vi "Add Leaves.vi"(0 "TreeControl in":refnum<vi>, 1 "Relative File Path":string, 3 "FileName In Hierarchy?":bool, 5 "Tree Parent Tags":string[](array[string]), 7 "Tree Items Created In":variant, 9 "Group/Channel Names":string[](array[string]), 11 "error in (no error)":errorcluster) -> (8 "Tree Items Created Out":variant, 15 "error out":errorcluster)   [LabVIEW 2017, in "XTree.xctl"]
doc: "Adds channels to the tree at the last hierarchical level, if they don't already exist in the Tree Items Created variant."
uses:
  <vilib>/addons/_NIFileIO/XTree/XTree.xctl
panel:
  # "The Tree Parent Tags parameter's dimensions\ncorrespond to Group and Channel."
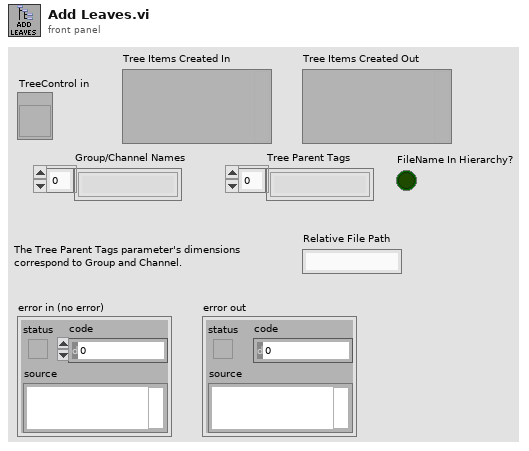
[diagram p1: front panel]
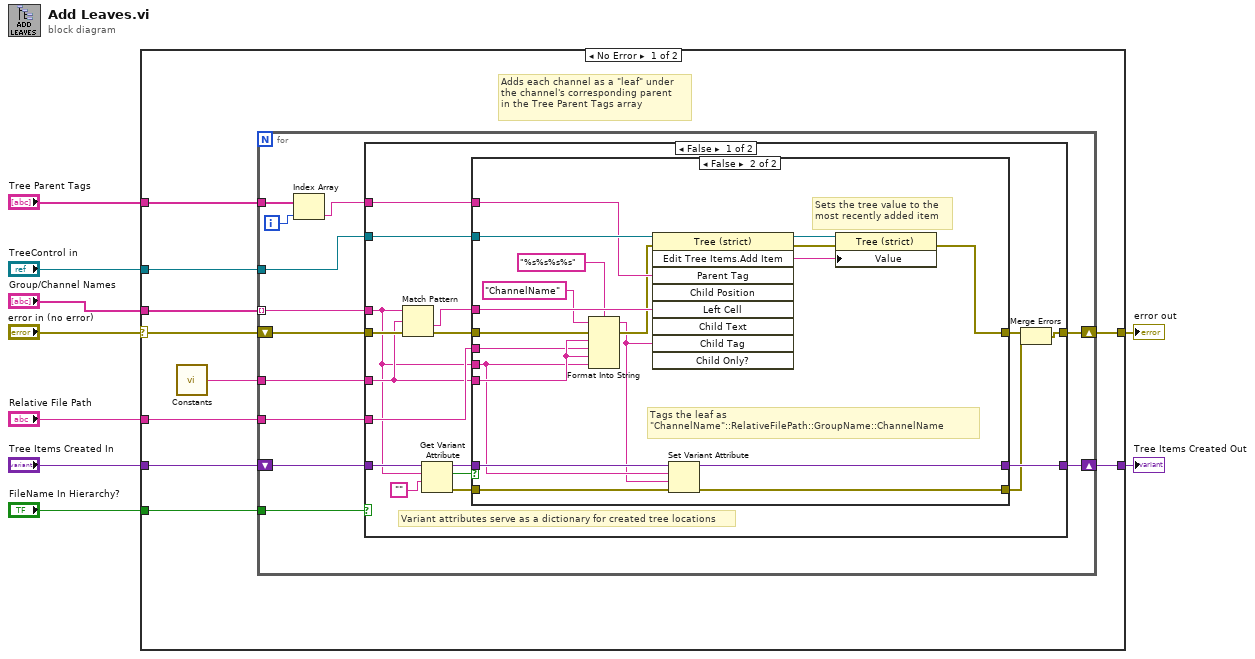
[diagram p0: block diagram]
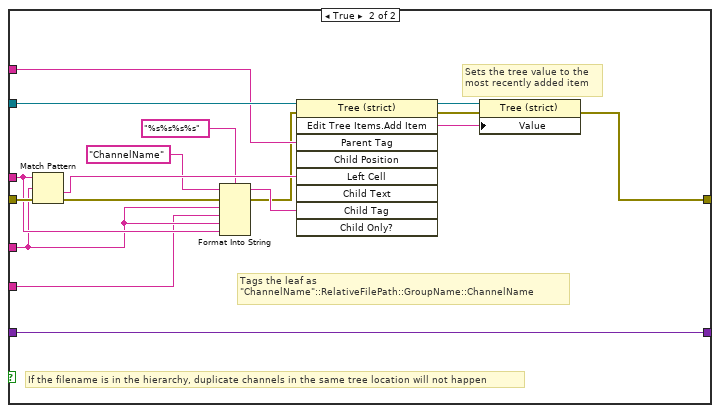
[diagram p3: hidden frame]
diagram:
  n1 = case shown="No Error" "error in (no error)" {
    selector: "error in (no error)" -> [w15 w86]
    tunnel: [w19 w86] -> w8
    tunnel: "Tree Items Created In" -> [w17 w87]
    tunnel: [w16 w87] -> w1
    tunnel: "FileName In Hierarchy?" -> [w14 _]
    tunnel: "Group/Channel Names" -> [w13 _]
    tunnel: "TreeControl in" -> [w12 _]
    tunnel: "Tree Parent Tags" -> [w11 _]
    tunnel: "Relative File Path" -> [w10 _]
    frame No Error {
      # "Adds each channel as a \"leaf\" under\nthe channel's corresponding parent\nin the Tree Parent Tags array"
      n2 = call <vilib>:"Constants.vi"() -> ("String Delimeter"=w18:string)  [unwired: 5 in]
      n3 = for {
        tunnel: w12 -> [w31]
        shift-right: [w29] -> w19
        shift-left: w15 -> [w30]
        tunnel: w18 -> [w25]
        tunnel: w11 -> [w22]
        tunnel: w13 -> [w28] mode=indexing
        shift-right: [w26] -> w16
        shift-left: w17 -> [w27]
        tunnel: w10 -> [w24]
        tunnel: w14 -> [w23]
        i -> [w21]
        n4 = Index Array(array=w22, index=w21) -> (element=w20:string)
        n5 = case shown="False" w23 {
          tunnel: w31 -> [w47 w85]
          tunnel: w30 -> [w46 w84]
          tunnel: [w35 w83] -> w29
          tunnel: w20 -> [w45 w82]
          tunnel: w28 -> [w38 w73]
          tunnel: w27 -> [w40 w74]
          tunnel: [w43 w74] -> w26
          tunnel: w25 -> [w41 w72]
          tunnel: w24 -> [w42 w71]
          frame False {
            # "Variant attributes serve as a dictionary for created tree locations"
            n6 = Match Pattern(string=w38, regular expression=w41) -> (after substring=w44:string)  [unwired: 1 in, 3 out]
            n7 = Get Variant Attribute(Variant=w40, name=w38, default value (empty Variant)="") -> (duplicate Variant=w39:variant, found=w37:bool, error out=w33:errorcluster)  [unwired: 1 in, 1 out]
            n8 = case shown="False" w37 {
              tunnel: w47 -> [_ w69]
              tunnel: w46 -> [w50 w65]
              tunnel: [w50 w62] -> w36
              tunnel: w45 -> [_ w68]
              tunnel: w44 -> [_ w67]
              tunnel: w38 -> [_ w55]
              tunnel: w39 -> [w49 w56]
              tunnel: [w49 w53] -> w43
              tunnel: w41 -> [_ w59]
              tunnel: w42 -> [_ w58]
              tunnel: [w48 w52] -> w34
              tunnel: w33 -> [w48 w51]
              frame True {
              }
              frame False {
                # "Sets the tree value to the most recently added item"
                # "Tags the leaf as \n\"ChannelName\"::RelativeFilePath::GroupName::ChannelName"
                n9 = Format Into String(format string="%s%s%s%s", initial string="ChannelName", error in=w65, w59, w58, w59, w55) -> (resulting string=w54:string, error out=w64:errorcluster)
                n10 = invoke class="Tree (strict)" method="Edit Tree Items.Add Item"(reference=w69, error in=w64, "Parent Tag"=w68, "Left Cell"=w67, "Child Tag"=w54) -> (reference out=w61:refnum<vi>, error out=w63:errorcluster, "Edit Tree Items:Add Item"=w60:string)  [unwired: 4 in, 6 out]
                n11 = Set Variant Attribute(Variant=w56, name=w55, value=w54, error in=w51) -> (Variant out=w53:variant, error out=w52:errorcluster)  [unwired: 1 out]
                n12 = property class="Tree (strict)"(reference=w61, error in=w63, "Value"=w60) -> (error out=w62:errorcluster)  [unwired: 1 out]
              }
            }
            n13 = Merge Errors(w36, w34) -> (w35:errorcluster)
          }
          frame True {
            # "Sets the tree value to the most recently added item"
            # "If the filename is in the hierarchy, duplicate channels in the same tree location will not happen"
            # "Tags the leaf as \n\"ChannelName\"::RelativeFilePath::GroupName::ChannelName"
            n14 = Match Pattern(string=w73, regular expression=w72) -> (after substring=w81:string)  [unwired: 1 in, 3 out]
            n15 = Format Into String(format string="%s%s%s%s", initial string="ChannelName", error in=w84, w72, w71, w72, w73) -> (resulting string=w79:string, error out=w78:errorcluster)
            n16 = invoke class="Tree (strict)" method="Edit Tree Items.Add Item"(reference=w85, error in=w78, "Parent Tag"=w82, "Left Cell"=w81, "Child Tag"=w79) -> (reference out=w76:refnum<vi>, error out=w77:errorcluster, "Edit Tree Items:Add Item"=w75:string)  [unwired: 4 in, 6 out]
            n17 = property class="Tree (strict)"(reference=w76, error in=w77, "Value"=w75) -> (error out=w83:errorcluster)  [unwired: 1 out]
          }
        }
      }
    }
    frame Error {
    }
  }
  "error out" <- w8
  "Tree Items Created Out" <- w1
